vi "PSTR-Progress Bar.vi"(0 "Data":T1, 2 "Action":enum16{"Init", "Seq", "Freq", "Level", "Hide"}(ring), 5 "Progress":refnum<vi>, 7 "Order Index":i32, 9 "Value Index":i32, 11 "error in (no error)":errorcluster) -> (15 "error out":errorcluster)   [LabVIEW 2020]
uses:
  Typedefs/PSTR-Data.ctl
  Typedefs/PSTR-Model Fit.ctl
  Typedefs/PSTR-Fit Parameters.ctl
panel:
  # "NF x NL x 2 x Npts"
  # "NF x NL x Npts"
  # "NF x NL"
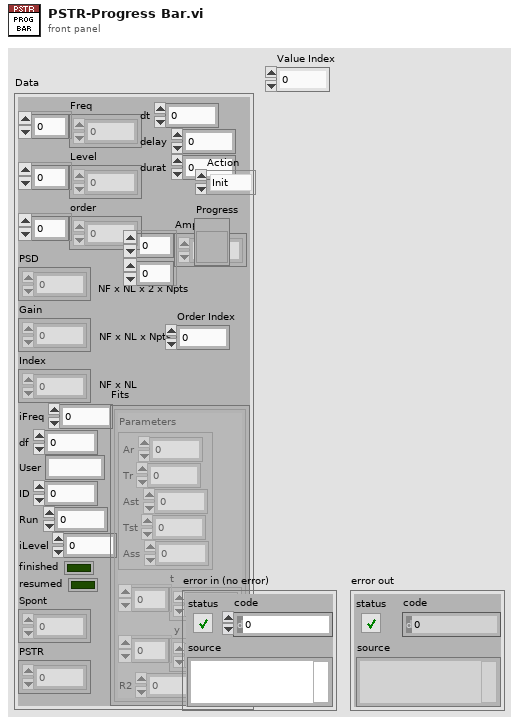
[diagram p1: front panel]
types:
  T1 = typedef "PSTR-Data.ctl" = cluster{"Freq":dbl[], "Level":dbl[], "order":i32[], "PSD":dbl[][][][], "Gain":dbl[][][], "Index":dbl[][], "iFreq":i32, "df":dbl, "User":string, "ID":i32, "Run":i32, "iLevel":i32, "finished":bool, "resumed":bool, "Spont":dbl[][], "PSTR":dbl[][][], "dt":dbl, "delay":dbl, "durat":dbl, "Fits":T2[][], "Amplitude":dbl[][]}
  T2 = typedef "PSTR-Model Fit.ctl" = cluster{"Parameters":T3, "t":dbl[], "y":dbl[], "R2":dbl}
  T3 = typedef "PSTR-Fit Parameters.ctl" = cluster{"Ar":dbl, "Tr":dbl, "Ast":dbl, "Tst":dbl, "Ass":dbl}
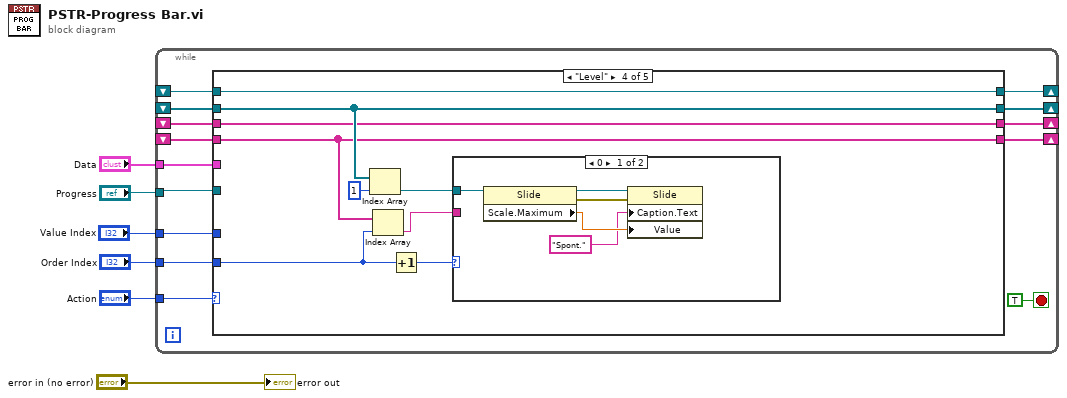
[diagram p0: block diagram]
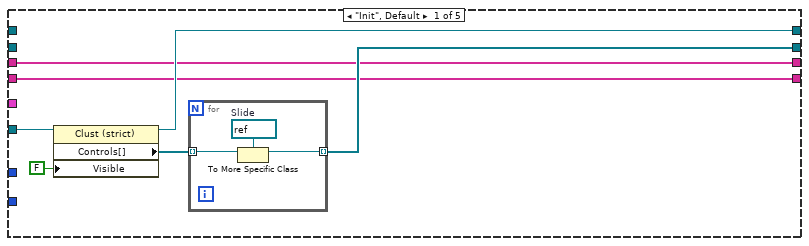
[diagram p2: hidden frame]
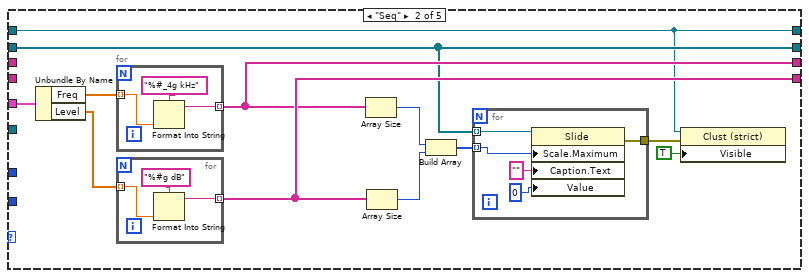
[diagram p3: hidden frame]
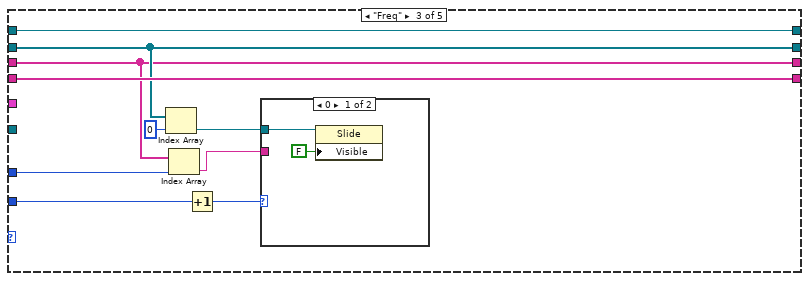
[diagram p4: hidden frame]
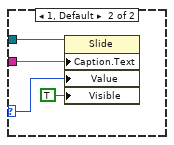
[diagram p5: hidden frame]
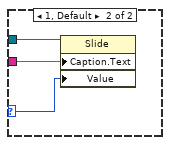
[diagram p6: hidden frame]
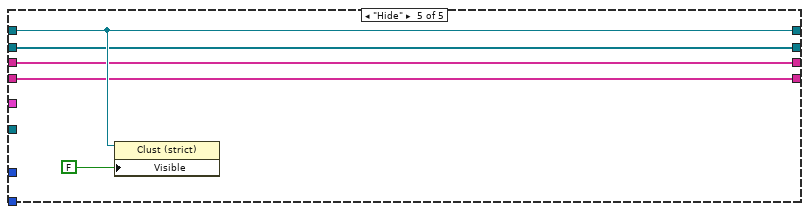
[diagram p7: hidden frame]
diagram:
  n1 = while {
    tunnel: "Progress" -> [w18]
    tunnel: "Action" -> [w19]
    shift-right: [w17] -> _
    shift-left: _ -> [w16]
    tunnel: "Data" -> [w15]
    shift-right: [w14] -> _
    shift-left: _ -> [w13]
    shift-right: [w11] -> _
    shift-left: _ -> [w9]
    shift-right: [w12] -> _
    shift-left: _ -> [w10]
    tunnel: "Order Index" -> [w8]
    tunnel: "Value Index" -> [w7]
    stop <- TRUE stop-if-true
    n2 = case shown="\"Level\"" w19 {
      tunnel: w18 -> [w27 _ _ _ _]
      tunnel: [w25 w32 w63 w78 w91] -> w17
      tunnel: w16 -> [_ w32 w63 w78 w91]
      tunnel: w15 -> [_ w42 _ _ _]
      tunnel: [w23 w34 w61 w77 w89] -> w14
      tunnel: w13 -> [_ w34 w61 w77 w89]
      tunnel: [w22 w38 w60 w76 w88] -> w12
      tunnel: [w21 w39 w62 w70 w87] -> w11
      tunnel: w10 -> [w22 _ w60 w76 w88]
      tunnel: w9 -> [w21 _ w62 w70 w87]
      tunnel: w8 -> [_ _ w57 w73 _]
      tunnel: w7 -> [_ _ w54 _ _]
      frame "Init", Default {
        n3 = property class="Clust (strict)"(reference=w27, "Visible"=FALSE) -> (reference out=w25:refnum<vi>, "Controls[]"=w26:refnum<vi>[])  [unwired: 1 in, 1 out]
        n4 = for {
          tunnel: w26 -> [w28] mode=indexing
          tunnel: [w29] -> w23 mode=indexing
          w30 = refnum<vi> refnum  # Slide
          n5 = To More Specific Class(target class=w30, reference=w28) -> (specific class reference=w29:refnum<vi>)  [unwired: 1 in, 1 out]
        }
      }
      frame "Seq" {
        n6 = Unbundle By Name(w42) -> ("Freq"=w41:dbl[], "Level"=w40:dbl[])
        n7 = for {
          tunnel: w41 -> [w53] mode=indexing
          tunnel: [w51] -> w38 mode=indexing
          n8 = Format Into String(format string="%#_4g kHz", w53) -> (resulting string=w51:string)  [unwired: 2 in, 1 out]
        }
        n9 = for {
          tunnel: w40 -> [w50] mode=indexing
          tunnel: [w48] -> w39 mode=indexing
          n10 = Format Into String(format string="%#g dB", w50) -> (resulting string=w48:string)  [unwired: 2 in, 1 out]
        }
        n11 = Array Size(array=w38) -> (size(s)=w37:i32)
        n12 = Array Size(array=w39) -> (size(s)=w36:i32)
        n13 = Build Array(w37, w36) -> (w35:i32[])
        n14 = for {
          tunnel: w35 -> [w46] mode=indexing
          tunnel: w34 -> [w47] mode=indexing
          tunnel: [w44] -> w33
          n15 = property class="Slide"(reference=w47, "Scale.Maximum"=w46, "Caption.Text"="", "Value"=0) -> (error out=w44:errorcluster)  [unwired: 1 in, 1 out]
        }
        n16 = property class="Clust (strict)"(reference=w32, error in=w33, "Visible"=TRUE) -> ()  [unwired: 2 out]
      }
      frame "Freq" {
        n17 = Index Array(array=w61, index=0) -> (element=w59:refnum<vi>)
        n18 = Index Array(array=w60, index=w54) -> (element=w58:string)
        n19 = Increment(x=w57) -> (x+1=w56:i32)
        n20 = case shown="0" w56 {
          selector: w56 -> [_ w67]
          tunnel: w59 -> [w65 w69]
          tunnel: w58 -> [_ w68]
          frame 0 {
            n21 = property class="Slide"(reference=w65, "Visible"=FALSE) -> ()  [unwired: 1 in, 2 out]
          }
          frame 1, Default {
            n22 = property class="Slide"(reference=w69, "Caption.Text"=w68, "Value"=w67, "Visible"=TRUE) -> ()  [unwired: 1 in, 2 out]
          }
        }
      }
      frame "Level" {
        n23 = Index Array(array=w77, index=1) -> (element=w75:refnum<vi>)
        n24 = Index Array(array=w70, index=w73) -> (element=w74:string)
        n25 = Increment(x=w73) -> (x+1=w72:i32)
        n26 = case shown="0" w72 {
          selector: w72 -> [_ w84]
          tunnel: w75 -> [w83 w86]
          tunnel: w74 -> [_ w85]
          frame 0 {
            n27 = property class="Slide"(reference=w83) -> (reference out=w82:refnum<vi>, error out=w81:errorcluster, "Scale.Maximum"=w80:dbl)  [unwired: 1 in]
            n28 = property class="Slide"(reference=w82, error in=w81, "Caption.Text"="Spont.", "Value"=w80) -> ()  [unwired: 2 out]
          }
          frame 1, Default {
            n29 = property class="Slide"(reference=w86, "Caption.Text"=w85, "Value"=w84) -> ()  [unwired: 1 in, 2 out]
          }
        }
      }
      frame "Hide" {
        n30 = property class="Clust (strict)"(reference=w91, "Visible"=FALSE) -> ()  [unwired: 1 in, 2 out]
      }
    }
  }
  "error out" <- "error in (no error)"
